vi "Read ActiveChannel.vi"(8 "error in (no error)":errorcluster, 11 "TektronixDPO_PhysicalDevice in":refnum<class "TektronixDPO_PhysicalDevice.lvclass">) -> (0 "error out":errorcluster, 2 "ActiveChannel":T2={"Channel"=1, "offset"=0.0, "verticalrange"=0.0, "Impedance"=0, "Probe Attenuation"=1.0, "Vertical Coupling"=1, "Bandwidth"=0, "Enabled"=FALSE} {"Bandwidth" items=["FULL", "250 MHz", "150 MHz", "20 MHz"]; "Vertical Coupling" items=["AC", "DC", "Ground"]; "Impedance" items=["1M", "75", "50"]; "Channel" items=["Channel 1", "Channel 2", "Channel 3", "Channel 4", "Math", "Reference 1", "Reference 2", "Reference 3", "Reference 4", "Bus 1", "Bus 2"]}, 3 "TektronixDPO_PhysicalDevice out":refnum<class "TektronixDPO_PhysicalDevice.lvclass">)   [LabVIEW 2013, in "TektronixDPO_PhysicalDevice.lvclass"]
uses:
  TektronixDPO_PhysicalDevice.lvclass
  shared/Typdefs/Choice80.ctl
  TektronixDPO_PhysicalDevice.lvclass/TektronixDPO_PhysicalDevice.ctl
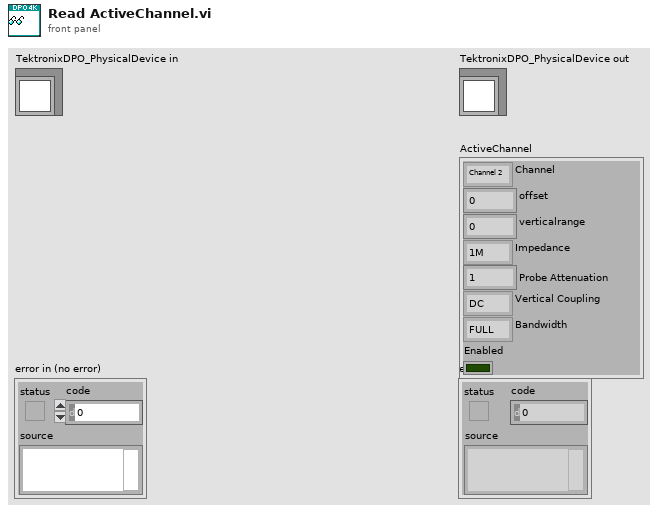
[diagram p1: front panel]
types:
  T1 = typedef "Choice80.ctl" = u16
  T2 = cluster{"Channel":T1, "offset":dbl, "verticalrange":dbl, "Impedance":u16, "Probe Attenuation":dbl, "Vertical Coupling":u16, "Bandwidth":u16, "Enabled":bool}
  T3 = typedef "Choice78.ctl" = enum16{"1M", "75", "50"}
  T4 = typedef "Choice11.ctl" = enum16{"AC", "DC", "Ground"}
  T5 = typedef "Choice79.ctl" = enum16{"FULL", "250 MHz", "150 MHz", "20 MHz"}
  T6 = cluster{"Channel":T1, "offset":dbl, "verticalrange":dbl, "Impedance":T3, "probeattenuation":dbl, "coupling":T4, "bandwidth":T5, "channelenabled":bool}
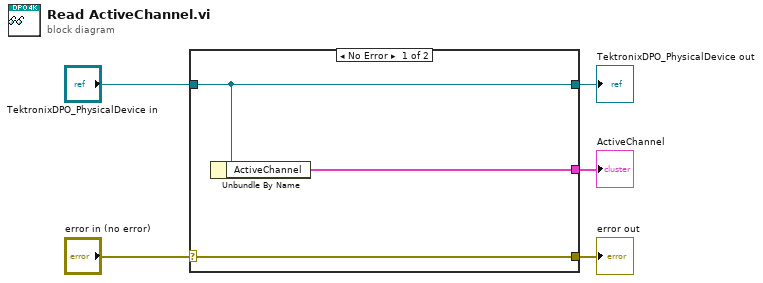
[diagram p0: block diagram]
diagram:
  n1 = case shown="No Error" "error in (no error)" {
    selector: "error in (no error)" -> [w8 w9]
    tunnel: [w8 w9] -> w4
    tunnel: [w7 w10] -> w2
    tunnel: "TektronixDPO_PhysicalDevice in" -> [w7 w10]
    tunnel: [w6 _] -> w1
    frame No Error {
      n2 = Unbundle By Name(w7) -> ("ActiveChannel"=w6:T6)
    }
    frame Error {
    }
  }
  "error out" <- w4
  "TektronixDPO_PhysicalDevice out" <- w2
  "ActiveChannel" <- w1
